vi "Taller 1 punto 3.vi"() -> ()   [LabVIEW 2017]
panel:
  out "Decremento":bool
  out "Incremento":bool
  in  "Decremento T":dbl(knob) scale=0.0..10.0
  in  "Incremento T":dbl(knob) scale=0.0..10.0
  in  "SELECTOR":bool
  in  "RATA DE T (°C/Seg)":dbl(knob) scale=1.0..10.0
  in  "Temp Mín":dbl
  in  "Temp Máx":dbl
  out "Sensor de Temperatura °C":dbl(slide) scale=0.0..200.0
  # "TALLER 1, PUNTO 3\nLUZ ANDREA JARAMILLO CASTILLO"
  # "DECREMENTAR"
  # "INCREMENTAR"
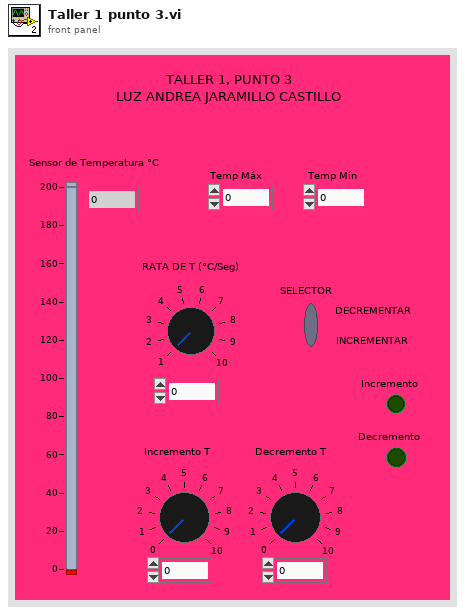
[diagram p1: front panel]
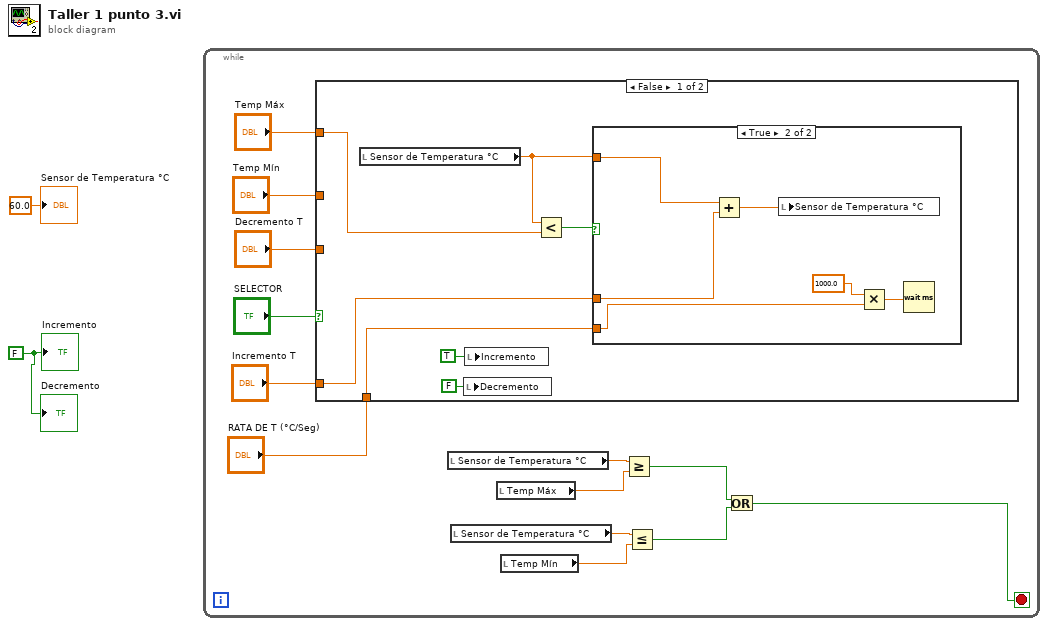
[diagram p0: block diagram]
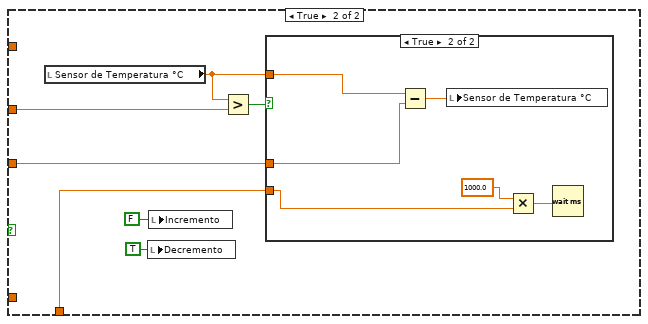
[diagram p3: hidden frame]
diagram:
  w1 = FALSE ("Incremento")
  n1 = while {
    stop <- w8 stop-if-true
    n2 = case shown="False" "SELECTOR" {
      tunnel: "Temp Mín" -> [_ w31]
      tunnel: "Decremento T" -> [_ w30]
      tunnel: "Temp Máx" -> [w18 _]
      tunnel: "Incremento T" -> [w17 _]
      tunnel: "RATA DE T (°C/Seg)" -> [w16 w29]
      frame False {
        n3 = local read "Sensor de Temperatura °C"() -> (w21:dbl)
        n4 = local write "Decremento"(FALSE ("Incremento")) -> ()
        n5 = local write "Incremento"(TRUE ("Incremento")) -> ()
        n6 = Less?(x=w21, y=w18) -> (x < y?=w22:bool)
        n7 = case shown="True" w22 {
          tunnel: w21 -> [_ w27]
          tunnel: w17 -> [_ w24]
          tunnel: w16 -> [_ w23]
          frame False {
          }
          frame True {
            n8 = Add(x=w27, y=w24) -> (x+y=w28:dbl)
            n9 = local write "Sensor de Temperatura °C"(w28) -> ()
            n10 = Multiply(x=1000.0, y=w23) -> (x*y=w25:dbl)
            n11 = Wait (ms)(milliseconds to wait=w25) -> ()  [unwired: 1 out]
          }
        }
      }
      frame True {
        n12 = local read "Sensor de Temperatura °C"() -> (w34:dbl)
        n13 = local write "Decremento"(TRUE ("Incremento")) -> ()
        n14 = local write "Incremento"(FALSE ("Incremento")) -> ()
        n15 = Greater?(x=w34, y=w31) -> (0:w35:bool)
        n16 = case shown="True" w35 {
          tunnel: w34 -> [_ w40]
          tunnel: w30 -> [_ w37]
          tunnel: w29 -> [_ w36]
          frame False {
          }
          frame True {
            n17 = Subtract(x=w40, y=w37) -> (x-y=w41:dbl)
            n18 = local write "Sensor de Temperatura °C"(w41) -> ()
            n19 = Multiply(x=1000.0, y=w36) -> (x*y=w39:dbl)
            n20 = Wait (ms)(milliseconds to wait=w39) -> ()  [unwired: 1 out]
          }
        }
      }
    }
    n21 = local read "Sensor de Temperatura °C"() -> (w14:dbl)
    n22 = local read "Sensor de Temperatura °C"() -> (w11:dbl)
    n23 = local read "Temp Máx"() -> (w13:dbl)
    n24 = local read "Temp Mín"() -> (w12:dbl)
    n25 = Greater Or Equal?(x=w14, y=w13) -> (x >= y?=w10:bool)
    n26 = Less Or Equal?(x=w11, y=w12) -> (x <= y?=w9:bool)
    n27 = Or(x=w10, y=w9) -> (x .or. y?=w8:bool)
  }
  "Sensor de Temperatura °C" <- 60.0 ("Sensor de Temperatura °C")
  "Decremento" <- w1
  "Incremento" <- w1
